vi "Meas Result Fill Freq Selector.vi"(2 "meas":T1={"swp cfg"={"N"=0, "R"=0, "f list"=[], "smpl delay"=0.0, "set delay"=0.0, "set delay np"=0.0, "meas root"=path "", "meas name"="", "meas a-index"=FALSE, "rnd sweep"=FALSE, "mode"=enum."Frequency", "swp mode"=enum."Linear", "avg"=0, "subrec"=0, "multi-freq"=FALSE}, "bridge"={"type"=enum."TWM client", "TWM"={"pipe name"="", "parameters"=[], "handle"=0, "fixed aper [s]"=0.0, "f-list [Hz]"=[], "discrete f-list"=FALSE, "unc mode"=enum."None", "unc mcc"=0, "unc first"=FALSE}, "last f"=0.0, "bias comp"={"bias type"=enum."dummy", "VISA"="", "Enable"=FALSE, "channel qu"=[], "channel Uinit"=[]}}, "src"={"type"=enum."Tektronix AFG3101C", "afg"={"VISA"="", "const"=0.0, "gen DC"=FALSE, "ext ref"=FALSE}, "cDAQ dds"={"device"="", "channels"=[], "mclk source"="", "mclk [Hz]"=0.0, "use ext mclk"=FALSE, "fs [Hz]"=0.0, "block [s]"=0.0, "buf [s]"=0.0, "task"="", "cmd queue"=refnum, "proc ref"=refnum, "smpl clock out"="/cDAQ3/PFI0", "export smpl clock"=FALSE, "DC ofs [V]"=[]}, "gain [V/A]"=1.0, "F5xxx session"={"VISA"="", "mode"=enum."AC voltage", "Earth on"=FALSE, "Ext ref lock"=FALSE}}, "results"=refnum} {"src"."cDAQ dds"."channels" min=0 step=1; "bridge"."TWM"."f-list [Hz]" format="%#_6p"; "swp cfg"."f list"."bias" format="%#_3p"; "swp cfg"."f list"."level" format="%#_3p"; "swp cfg"."f list"."fs [Hz]" format="%#_5p"; "swp cfg"."f list"."time [s]" format="%#_3p"; "swp cfg"."f list"."f/fs" format="%#_3p"; "swp cfg"."f list"."periods" format="%#_3f"; "swp cfg"."f list"."f [Hz]" format="%#_5p"}, 3 "results data":T19, 4 "res fid":refnum<vi>) -> (0 "freq filter (NaN: no filter)":dbl, 1 "freq index (default: 0)":u16)   [LabVIEW 2013]
doc: "Fills list of frequencies selector based on available sweep spots cout available in result data."
uses:
  Meas Results.ctl
  bridge/Bridge Frequency Readings Data.ctl
  drivers/TWM client/Meas Proc QWTB Spectrum Data.ctl
  meas session.ctl
  Meas Sweep Config.ctl
  Meas Freq Info.ctl
  meas_swp_mode.ctl
  meas_sweep_flist_mode.ctl
  bridge/Bridge Session.ctl
  bridge/Bridge Type.ctl
  drivers/TWM client/TWM Session.ctl
  drivers/TWM client/TWM parameters.ctl
  drivers/TWM client/Meas Proc QWTB Uncertainty Mode.ctl
  bridge/Bridge Bias Session.ctl
  bridge/Bridge Bias Type.ctl
  source/Source Session.ctl
  source/Source Type.ctl
  drivers/AFG3101C/AFG3101C Session.ctl
  drivers/cDAQ DDS/cDAQ DDS Session.ctl
  drivers/cDAQ DDS/cDAQ DDS Setup.ctl
  drivers/Fluke 5XXX/top_lev/F5xxx_session.ctl
  drivers/Fluke 5XXX/top_lev/F5xxx_output_mode.ctl
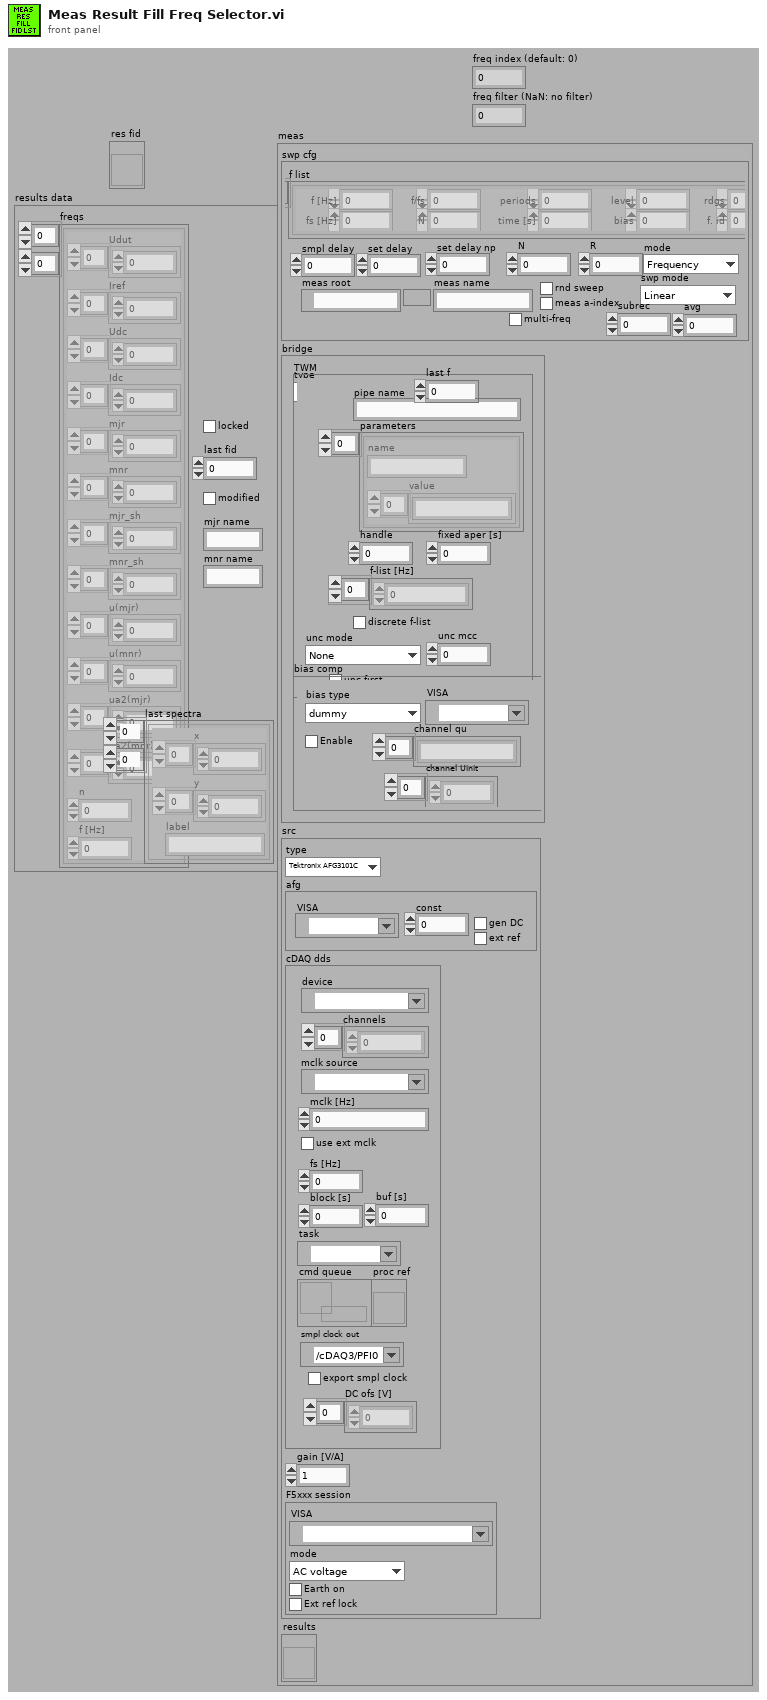
[diagram p1: front panel]
types:
  T1 = typedef "meas session.ctl" = cluster{"swp cfg":T2, "bridge":T6, "src":T13, "results":refnum<vi>}
  T2 = typedef "Meas Sweep Config.ctl" = cluster{"N":i32, "R":i32, "f list":T3[], "smpl delay":dbl, "set delay":dbl, "set delay np":dbl, "meas root":path, "meas name":string, "meas a-index":bool, "rnd sweep":bool, "mode":T4, "swp mode":T5, "avg":i32, "subrec":i32, "multi-freq":bool}
  T3 = typedef "Meas Freq Info.ctl" = cluster{"f [Hz]":dbl, "periods":dbl, "f/fs":dbl, "time [s]":dbl, "fs [Hz]":dbl, "N":i32, "level":dbl, "bias":dbl, "rdgs":i32, "f. id":i32}
  T4 = typedef "meas_swp_mode.ctl" = enum16{"Frequency", "Level", "Bias"}
  T5 = typedef "meas_sweep_flist_mode.ctl" = enum16{"Linear", "Log10"}
  T6 = typedef "Bridge Session.ctl" = cluster{"type":T7, "TWM":T8, "last f":dbl, "bias comp":T11}
  T7 = typedef "Bridge Type.ctl" = enum16{"TWM client", "dummy"}
  T8 = typedef "TWM Session.ctl" = cluster{"pipe name":string, "parameters":T9[], "handle":i32, "fixed aper [s]":dbl, "f-list [Hz]":dbl[], "discrete f-list":bool, "unc mode":T10, "unc mcc":i32, "unc first":bool}
  T9 = typedef "TWM parameters.ctl" = cluster{"name":string, "value":string[]}
  T10 = typedef "Meas Proc QWTB Uncertainty Mode.ctl" = enum16{"None", "GUF", "Monte Carlo"}
  T11 = typedef "Bridge Bias Session.ctl" = cluster{"bias type":T12, "VISA":refnum<visa-resource-name>, "Enable":bool, "channel qu":string[], "channel Uinit":dbl[]}
  T12 = typedef "Bridge Bias Type.ctl" = enum16{"dummy", "CMI LiBbias V1.0"}
  T13 = typedef "Source Session.ctl" = cluster{"type":T14, "afg":T15, "cDAQ dds":T16, "gain [V/A]":dbl, "F5xxx session":T17}
  T14 = typedef "Source Type.ctl" = enum16{"Tektronix AFG3101C", "cDAQ DAC", "Fluke 5xxx", "Agilent 33120A", "dummy"}
  T15 = typedef "AFG3101C Session.ctl" = cluster{"VISA":refnum<visa-resource-name>, "const":dbl, "gen DC":bool, "ext ref":bool}
  T16 = typedef "cDAQ DDS Session.ctl" = cluster{"device":tag, "channels":i32[], "mclk source":tag, "mclk [Hz]":dbl, "use ext mclk":bool, "fs [Hz]":dbl, "block [s]":dbl, "buf [s]":dbl, "task":refnum<k21>, "cmd queue":refnum<queue>, "proc ref":refnum<vi>, "smpl clock out":tag, "export smpl clock":bool, "DC ofs [V]":dbl[]}
  T17 = typedef "F5xxx_session.ctl" = cluster{"VISA":refnum<visa-resource-name>, "mode":T18, "Earth on":bool, "Ext ref lock":bool}
  T18 = typedef "F5xxx_output_mode.ctl" = enum16{"AC voltage", "AC current"}
  T19 = typedef "Meas Results.ctl" = cluster{"freqs":T20[][], "locked":bool, "last fid":i32, "modified":bool, "mjr name":string, "mnr name":string, "last spectra":T21[][]}
  T20 = typedef "Bridge Frequency Readings Data.ctl" = cluster{"Udut":dbl[], "Iref":dbl[], "Udc":dbl[], "Idc":dbl[], "mjr":dbl[], "mnr":dbl[], "mjr_sh":dbl[], "mnr_sh":dbl[], "u(mjr)":dbl[], "u(mnr)":dbl[], "ua2(mjr)":dbl[], "ua2(mnr)":dbl[], "n":i32, "f [Hz]":dbl}
  T21 = typedef "Meas Proc QWTB Spectrum Data.ctl" = cluster{"x":sgl[], "y":sgl[], "label":string}
  T22 = enum8{"Enabled", "Disabled", "Disabled and Grayed Out"}
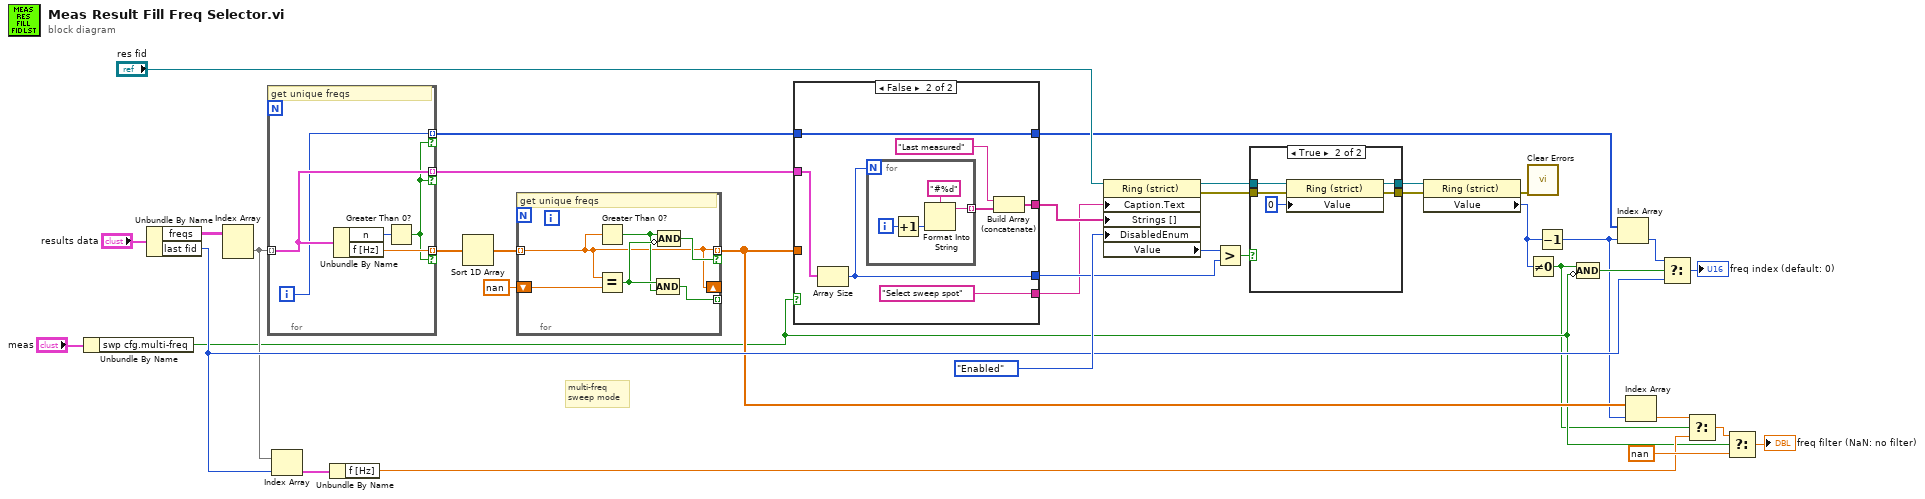
[diagram p0: block diagram]
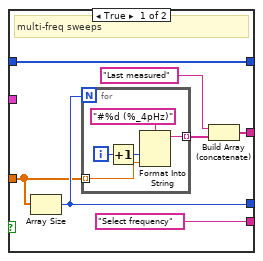
[diagram p2: hidden frame]
diagram:
  # "multi-freq\nsweep mode"
  n1 = Unbundle By Name("meas") -> ("swp cfg.multi-freq"=w10:bool)
  n2 = Unbundle By Name("results data") -> ("freqs"=w32:T20[][], "last fid"=w22:i32)
  n3 = Index Array(array=w32) -> (element=w20:T20[])  [unwired: 2 in]
  n4 = for {
    tunnel: w20 -> [w40] mode=indexing
    tunnel: [w42] -> w15 mode=indexing if=w38
    tunnel: [w40] -> w5 mode=indexing if=w38
    tunnel: [w39] -> w4 mode=indexing if=w38
    i -> [w39]
    # "get unique freqs"
    n5 = Unbundle By Name(w40) -> ("n"=w41:i32, "f [Hz]"=w42:dbl)
    n6 = Greater Than 0?(x=w41) -> (x > 0?=w38:bool)
  }
  n7 = Index Array(array=w20, index=w22) -> (element=w21:T20)
  n8 = Unbundle By Name(w21) -> ("f [Hz]"=w18:dbl)
  n9 = Sort 1D Array(array=w15) -> (sorted array=w12:dbl[])
  n10 = for {
    tunnel: w12 -> [w43] mode=indexing
    shift-right: [w43] -> _
    shift-left: nan ("f [Hz]") -> [w48]
    tunnel: [w44] -> _ mode=indexing
    tunnel: [w43] -> w13 mode=indexing if=w47
    # "get unique freqs"
    n11 = Greater Than 0?(x=w43) -> (x > 0?=w45:bool)
    n12 = Equal?(x=w43, y=w48) -> (x = y?=w46:bool)
    n13 = Compound Arithmetic op=AND(w46, w45) -> (w44:bool)
    n14 = Compound Arithmetic op=AND(w45, invert w46) -> (w47:bool)
  }
  n15 = case shown="False" w10 {
    tunnel: [w55 w67] -> w26
    tunnel: w13 -> [w54 _]
    tunnel: [w53 w66] -> w25
    tunnel: w5 -> [_ w63]
    tunnel: ["Select frequency" "Select sweep spot"] -> w17
    tunnel: w4 -> [w49 w61]
    tunnel: [w49 w61] -> w2
    frame True {
      # "multi-freq sweeps"
      n16 = Array Size(array=w54) -> (size(s)=w55:i32)
      n17 = for {
        N: w55 -> [_]
        tunnel: [w57] -> w52 mode=indexing
        tunnel: w54 -> [w56] mode=indexing
        i -> [w60]
        n18 = Increment(x=w60) -> (x+1=w59:i32)
        n19 = Format Into String(format string="#%d (%_4pHz)", w59, w56) -> (resulting string=w57:string)  [unwired: 2 in, 1 out]
      }
      n20 = Build Array (concatenate)("Last measured", w52) -> (w53:string[])
    }
    frame False {
      n21 = Array Size(array=w63) -> (size(s)=w67:i32)
      n22 = for {
        N: w67 -> [_]
        tunnel: [w68] -> w65 mode=indexing
        i -> [w71]
        n23 = Increment(x=w71) -> (x+1=w70:i32)
        n24 = Format Into String(format string="#%d", w70) -> (resulting string=w68:string)  [unwired: 2 in, 1 out]
      }
      n25 = Build Array (concatenate)("Last measured", w65) -> (w66:string[])
    }
  }
  n26 = property class="Ring (strict)"(reference="res fid", "Caption.Text"=w17, "Strings []"=w25, "DisabledEnum"=T22."Enabled" ("Disabled")) -> (reference out=w27:refnum<vi>, error out=w28:errorcluster, "Value"=w30:u16)  [unwired: 1 in]
  n27 = Greater?(x=w30, y=w26) -> (0:w29:bool)
  n28 = case shown="True" w29 {
    tunnel: w28 -> [w73 w78]
    tunnel: w27 -> [w72 w77]
    tunnel: [w73 w75] -> w35
    tunnel: [w72 w74] -> w34
    frame False {
    }
    frame True {
      n29 = property class="Ring (strict)"(reference=w77, error in=w78, "Value"=u16 0) -> (reference out=w74:refnum<vi>, error out=w75:errorcluster)
    }
  }
  n30 = property class="Ring (strict)"(reference=w34, error in=w35) -> (error out=w33:errorcluster, "Value"=w23:u16)  [unwired: 1 out]
  n31 = call <vilib>:"Clear Errors.vi"("error in (no error)"=w33) -> ()  [unwired: 6 in, 1 out]
  n32 = Not Equal To 0?(x=w23) -> (x != 0?=w9:bool)
  n33 = Decrement(x=w23) -> (x-1=w1:u16)
  n34 = Compound Arithmetic op=AND(w9, invert w10) -> (w11:bool)
  n35 = Index Array(array=w2, index=w1) -> (element=w3:i32)
  n36 = Index Array(array=w13, index=w1) -> (element=w7:dbl)
  n37 = Select(t=w3, s=w11, f=w22) -> (s? t:f=→"freq index (default: 0)":i32)
  n38 = Select(t=w7, s=w9, f=w18) -> (s? t:f=w6:dbl)
  n39 = Select(t=w6, s=w10, f=nan) -> (s? t:f=→"freq filter (NaN: no filter)":dbl)
